vi "Transfer.Config to Runtime.vi"(8 "error in (no error)":errorcluster, 10 "Transfer Configuration":refnum<class "Configuration.Transfer.lvclass">, 11 "Device Ref in":T1=18446744073709551615 format="%.0x") -> (0 "error out":errorcluster, 2 "Transfer Runtime":refnum<class "Runtime.Transfer.lvclass">, 3 "Device Ref out":T1=18446744073709551615 format="%.0x")   [LabVIEW 2016, in "Data Sharing Framework.Runtime.lvlib"]
uses:
  Data Sharing Framework.Runtime.lvlib
  <vilib>/NI Veristand/Custom Device API/Custom Device Item Ref.ctl
  Classes/Configuration.Transfer/Configuration.Transfer.lvclass
  Classes/Runtime/Transfer/Runtime.Transfer.lvclass
  Classes/Configuration.Transfer/Configuration.Transfer.lvclass/Configuration.Transfer.ctl
  Classes/Runtime/Transfer/Runtime.Transfer.lvclass/Runtime.Transfer.ctl
  Classes/Configuration.Channel/Configuration.Channel.lvclass
  <vilib>/NI VeriStand/Custom Device API/Custom Device API.lvlib
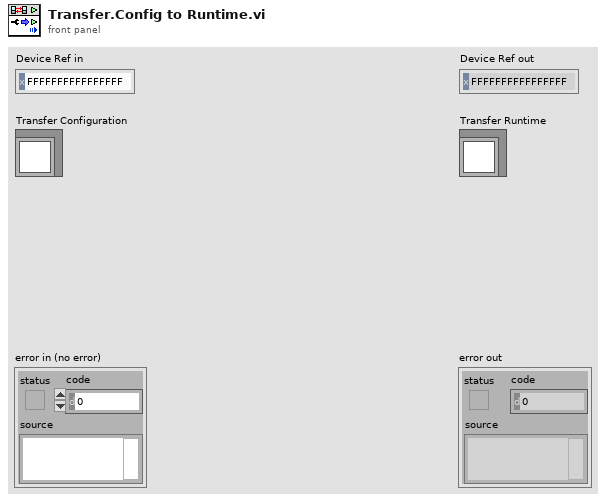
[diagram p1: front panel]
types:
  T1 = typedef "Custom Device API.lvlib/Custom Device Item Ref.ctl" = u64
  T2 = typedef "Custom Device API.lvlib/Data Access Type.ctl" = enum16{"Read", "Write"}
  T3 = typedef "Transfer Config.ctl" = cluster{"byte order":enum16{"big-endian, network order", "native, host order", "little-endian"}, "direction":T4, "decimation factors":T5}
  T4 = typedef "Transfer Direction.ctl" = enum16{"Transmit", "Receive"}
  T5 = typedef "Decimation Factors.ctl" = cluster{"decimation":u16, "offset":u16}
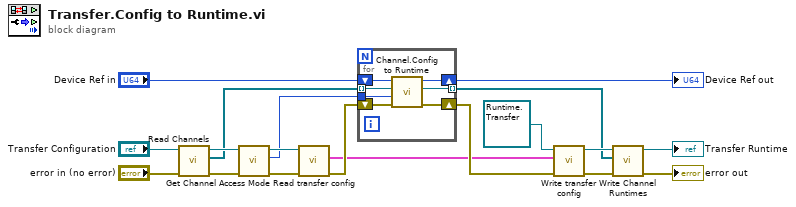
[diagram p0: block diagram]
diagram:
  n1 = call "Read Channels.vi"("error in (no error)"="error in (no error)", "Configuration.Transfer in"="Transfer Configuration") -> ("error out"=w13:errorcluster, "Channels"=w11:refnum<class "Configuration.Channel.lvclass">[], "Configuration.Transfer out"=w12:refnum<class "Configuration.Transfer.lvclass">)  [unwired: 7 in]
  n2 = call "Get Channel Access Mode.vi"("error in (no error)"=w13, "Transfer Configuration in"=w12) -> ("error out"=w9:errorcluster, "access"=w8:T2, "Transfer Configuration out"=w10:refnum<class "Configuration.Transfer.lvclass">)  [unwired: 7 in]
  n3 = call "Read transfer config.vi"("error in (no error)"=w9, "Configuration.Transfer in"=w10) -> ("error out"=w7:errorcluster, "transfer config"=w5:T3)  [unwired: 7 in, 1 out]
  n4 = for {
    tunnel: w11 -> [w26] mode=indexing
    tunnel: [w25] -> w3 mode=indexing
    shift-right: [w24] -> w6
    shift-left: w7 -> [w23]
    tunnel: w8 -> [w22]
    shift-right: [w20] -> w18
    shift-left: "Device Ref in" -> [w21]
    n5 = call "Channel.Config to Runtime.vi"("error in (no error)"=w23, "access"=w22, "Channel Configuration"=w26, "Device Ref in"=w21) -> ("error out"=w24:errorcluster, "Channel Runtime"=w25:refnum<class "Runtime.Channel.lvclass">, "Device Ref out"=w20:T1)  [unwired: 5 in]
  }
  "Device Ref out" <- w18
  n6 = call "Write transfer config.vi"("error in (no error)"=w6, "transfer config"=w5, "Runtime.Transfer in"=refnum<class "Runtime.Transfer.lvclass"> refnum ("Transfer Runtime")) -> ("error out"=w4:errorcluster, "Runtime.Transfer out"=w16:refnum<class "Runtime.Transfer.lvclass">)  [unwired: 7 in]
  n7 = call "Write Channel Runtimes.vi"("error in (no error)"=w4, "Channel Runtimes"=w3, "Runtime.Transfer in"=w16) -> ("error out"=→"error out":errorcluster, "Runtime.Transfer out"=→"Transfer Runtime":refnum<class "Runtime.Transfer.lvclass">)  [unwired: 7 in]
